vi "Handle SSE Request.vi"(8 "error in (no error)":errorcluster, 10 "Request":refnum<class "Request.lvclass">, 11 "SSE Handler in":refnum<class "SSE Handler.lvclass">) -> (0 "error out":errorcluster, 1 "Response":refnum<class "Response.lvclass">, 2 "SSE Manager":refnum<class "SSE Manager.lvclass">, 3 "SSE Handler out":refnum<class "SSE Handler.lvclass">, 5 "Last Event ID":string)   [LabVIEW 2020, in "HTTP Server.lvlib" / "SSE Handler.lvclass"]
uses:
  SSE Handler.lvclass
  lv-http-util/HTTP Utils/Request/Request.lvclass
  lv-http-util/HTTP Utils/Response/Response.lvclass
  SSE Manager/SSE Manager.lvclass
  SSE Handler.lvclass/SSE Handler.ctl
  lv-uri/URI/URI/URI.lvclass
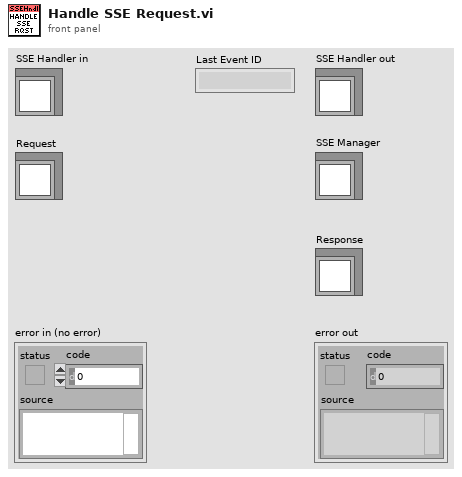
[diagram p1: front panel]
types:
  T1 = typedef "HTTP Server.lvlib/Server Sent Events Data.ctl" = cluster{"Resources":map{string, refnum<class "SSE Manager.lvclass">}}
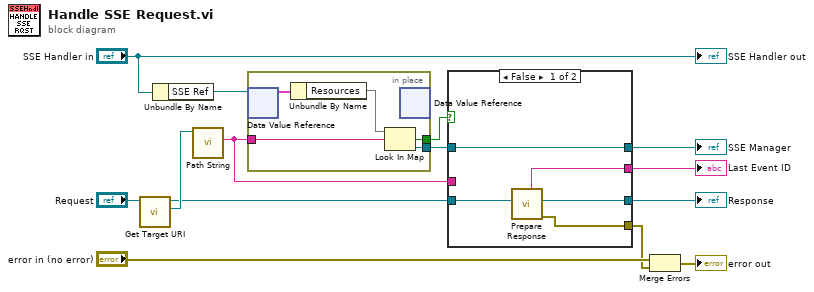
[diagram p0: block diagram]
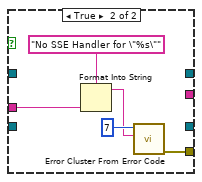
[diagram p2: hidden frame]
diagram:
  n1 = call "Get Target URI.vi"("Request in"="Request") -> ("Target URI"=w13:refnum<class "URI.lvclass">, "Request out"=w5:refnum<class "Request.lvclass">)  [unwired: 8 in, 1 out]
  n2 = Unbundle By Name("SSE Handler in") -> ("SSE Ref"=w10:refnum<data-value>)
  n3 = call "Path String.vi"("URI in"=w13) -> ("Path String"=w7:string)  [unwired: 9 in, 1 out]
  n4 = in-place {
    in-place-border: w7 -> [w18]
    in-place-border: [w17] -> w9
    in-place-border: [w15] -> w8
    n5 = in-place-dvr #1(w10) -> (w19:T1)  [unwired: 1 out]
    n6 = Unbundle By Name(w19) -> ("Resources"=w16:map{string, refnum<class "SSE Manager.lvclass">})
    n7 = Look In Map(map=w16, key=w18) -> (key not found?=w17:bool, value=w15:refnum<class "SSE Manager.lvclass">)  [unwired: 1 in]
    n8 = in-place-dvr #1() -> ()  [unwired: 1 in, 2 out]
  }
  n9 = case shown="False" w9 {
    tunnel: w8 -> [w24 _]
    tunnel: w7 -> [_ w27]
    tunnel: [w22 w25] -> w2
    tunnel: [w24 _] -> w6
    tunnel: w5 -> [w23 _]
    tunnel: [w21 _] -> w4
    tunnel: [w20 _] -> w1
    frame False {
      n10 = call "Prepare Response.vi"("Request"=w23) -> ("error out"=w22:errorcluster, "Response"=w21:refnum<class "Response.lvclass">, "Last Event ID"=w20:string)  [unwired: 8 in]
    }
    frame True {
      n11 = Format Into String(format string="No SSE Handler for \"%s\"", w27) -> (resulting string=w26:string)  [unwired: 2 in, 1 out]
      n12 = call <vilib>:"Error Cluster From Error Code.vi"("error message (\"\")"=w26, "error code (0)"=7) -> ("error out"=w25:errorcluster)  [unwired: 7 in]
    }
  }
  "Response" <- w4
  "SSE Manager" <- w6
  "Last Event ID" <- w1
  n13 = Merge Errors("error in (no error)", w2) -> (→"error out":errorcluster)
  "SSE Handler out" <- "SSE Handler in"
